vi "Get Item Property (Dependent File).vi"(8 "error in (no error)":errorcluster, 10 "Property Name":string, 11 "Item Ref in":T2 format="%.0x") -> (0 "error out":errorcluster, 2 "Path":path, 3 "Item Ref out":T2 format="%.0x", 4 "Found":bool, 5 "OptionalInfo":T1)   [LabVIEW 2020, in "Custom Device Offline API.lvlib"]
uses:
  <vilib>/NI VeriStand/Custom Device Offline API/Custom Device Offline API.lvlib
  <vilib>/NI VeriStand/Custom Device API/Custom Device Item Ref.ctl
  <vilib>/NI VeriStand/Custom Device API/Dependent File Optional Info.ctl
  NationalInstruments.VeriStand.SystemDefinitionAPI
  <vilib>/NI VeriStand/Custom Device API/Custom Device API.lvlib
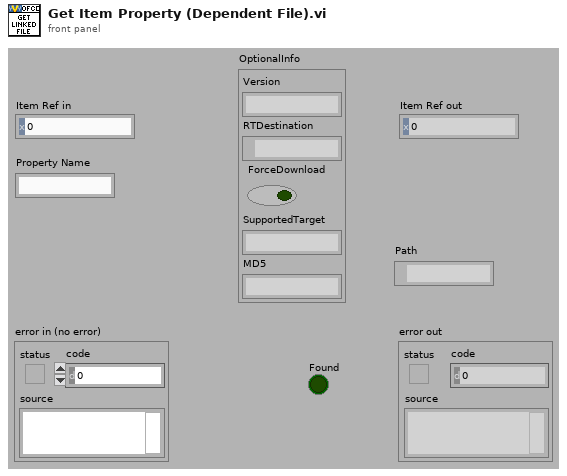
[diagram p1: front panel]
types:
  T1 = typedef "Custom Device API.lvlib/Dependent File Optional Info.ctl" = cluster{"Version":string, "RTDestination":path, "ForceDownload":bool, "SupportedTarget":string, "MD5":string}
  T2 = typedef "Custom Device API.lvlib/Custom Device Item Ref.ctl" = u64
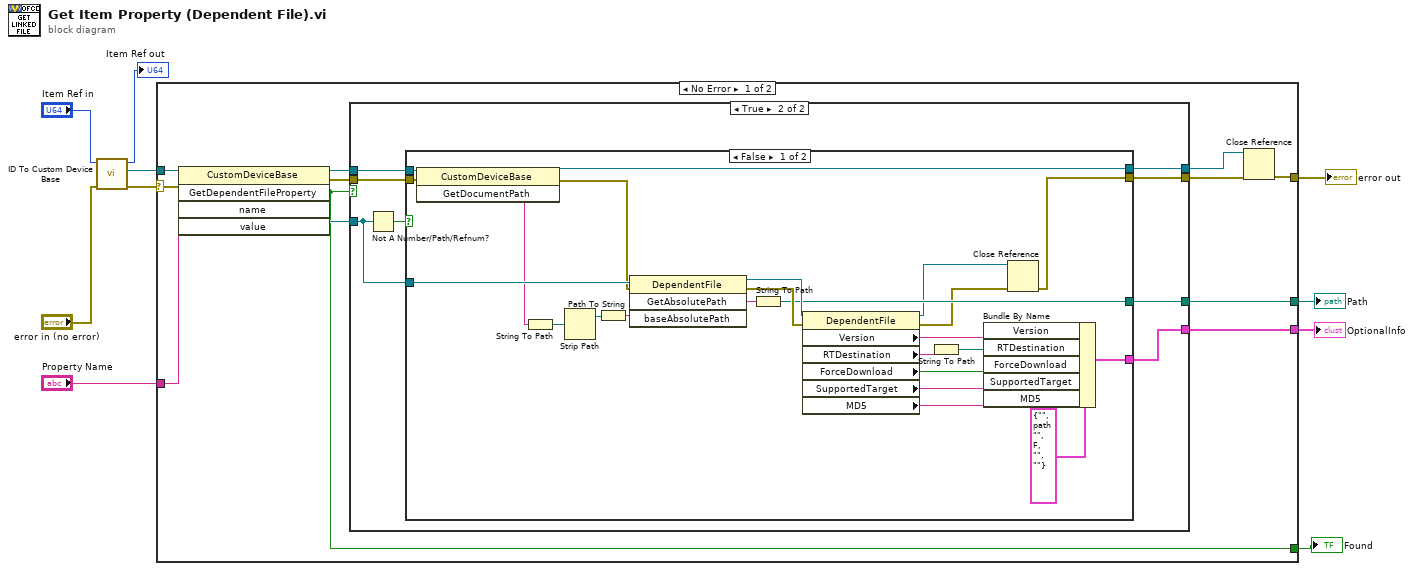
[diagram p0: block diagram]
diagram:
  n1 = call <vilib>:"ID To Custom Device Base.vi"("error in (no error)"="error in (no error)", "ID in"="Item Ref in") -> ("error out"=w9:errorcluster, "BaseNode"=w8:refnum<k24>, "ID out"=→"Item Ref out":u64)  [unwired: 7 in]
  n2 = case shown="No Error" w9 {
    selector: w9 -> [w16 w59]
    tunnel: w8 -> [w17 _]
    tunnel: [w20 w59] -> w2
    tunnel: [w19 _] -> w3
    tunnel: [w18 _] -> w1
    tunnel: "Property Name" -> [w15 _]
    tunnel: [w11 _] -> w4
    frame No Error {
      n3 = invoke class="CustomDeviceBase" method="GetDependentFileProperty"(reference=w17, error in=w16, "name"=w15) -> (reference out=w12:refnum<k24>, error out=w13:errorcluster, "GetDependentFileProperty"=w11:bool, "value"=w14:refnum<k24>)  [unwired: 2 in, 1 out]
      n4 = case shown="True" w11 {
        tunnel: [w23 w31] -> w22
        tunnel: [w24 w30] -> w21
        tunnel: [_ w29] -> w19
        tunnel: [_ w28] -> w18
        tunnel: w14 -> [_ w27]
        tunnel: w13 -> [w23 w26]
        tunnel: w12 -> [w24 w25]
        frame False {
        }
        frame True {
          n5 = Not A Number/Path/Refnum?(number/path/refnum=w27) -> (NaN/Path/Refnum?=w32:bool)
          n6 = case shown="False" w32 {
            tunnel: w25 -> [w56 w58]
            tunnel: w26 -> [w55 w57]
            tunnel: [w51 w57] -> w31
            tunnel: [w50 w58] -> w30
            tunnel: w27 -> [w54 _]
            tunnel: [w45 _] -> w29
            tunnel: [w48 _] -> w28
            frame False {
              n7 = invoke class="CustomDeviceBase" method="GetDocumentPath"(reference=w56, error in=w55) -> (reference out=w50:refnum<k24>, error out=w53:errorcluster, "GetDocumentPath"=w34:string)  [unwired: 1 in]
              n8 = String To Path(string=w34) -> (path=w36:path)
              n9 = Strip Path(path=w36) -> (stripped path=w35:path)  [unwired: 1 out]
              n10 = Path To String(path=w35) -> (string=w33:string)
              n11 = invoke class="DependentFile" method="GetAbsolutePath"(reference=w54, error in=w53, "baseAbsolutePath"=w33) -> (reference out=w47:refnum<k24>, error out=w46:errorcluster, "GetAbsolutePath"=w52:string)  [unwired: 1 in, 1 out]
              n12 = String To Path(string=w52) -> (path=w45:path)
              n13 = property class="DependentFile"(reference=w47, error in=w46) -> (reference out=w39:refnum<k24>, error out=w38:errorcluster, "Version"=w44:string, "RTDestination"=w43:string, "ForceDownload"=w41:bool, "SupportedTarget"=w40:string, "MD5"=w37:string)
              n14 = String To Path(string=w43) -> (path=w42:path)
              n15 = Bundle By Name(cluster=T1 {"Version"="", "RTDestination"=path "", "ForceDownload"=FALSE, "SupportedTarget"="", "MD5"=""} ("OptionalInfo"), "Version"=w44, "RTDestination"=w42, "ForceDownload"=w41, "SupportedTarget"=w40, "MD5"=w37) -> (w48:T1)
              n16 = Close Reference(reference=w39, error in (no error)=w38) -> (error out=w51:errorcluster)
            }
            frame True {
            }
          }
        }
      }
      n17 = Close Reference(reference=w21, error in (no error)=w22) -> (error out=w20:errorcluster)
    }
    frame Error {
    }
  }
  "error out" <- w2
  "Path" <- w3
  "Found" <- w4
  "OptionalInfo" <- w1
